vi "Keithley 2400 - Controle Fonte.vi"() -> ()   [LabVIEW 2011]
uses:
  <vilib>/Utility/file.llb/Write To Spreadsheet File (DBL).vi
panel:
  out "XY Graph":T1(graph)
  in  "VoltVector":dbl[](array[numeric])
  out "V(log)xI(log)":cluster{"Y":dbl[], "Y":dbl[]}[](graph)
  in  "Arquivo:":path=path "c:/dados.txt"
  in  "Corrente início:":dbl
  in  "CurrVector":dbl[](array[numeric])
  out "VxI":cluster{"Y":dbl[], "Y":dbl[]}[](graph)
  out "Corrente:":dbl
  out "Tensão:":dbl
  in  "Corrente limite (A):":dbl=2e-06
  in  "Porta Keithley:":refnum<visa-resource-name>="COM5"
  in  "Tensão passo (V):":dbl=1.0
  in  "Tensão final (V):":dbl=5.0
  in  "Tensão inicial (V):":dbl=1.0 caption="Tensão início:"
  in  "Medir":bool
  in  "Número de medidas:":i32=5
  in  "stop":bool
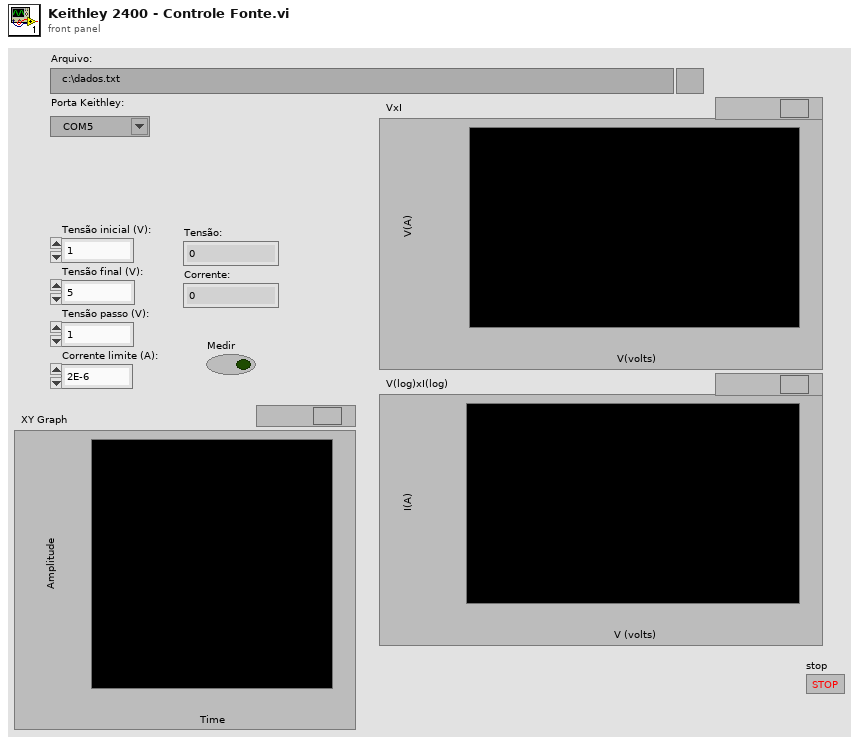
[diagram p1: front panel]
types:
  T1 = cluster{"VoltVector":dbl[], "CurrVector":dbl[]}[]
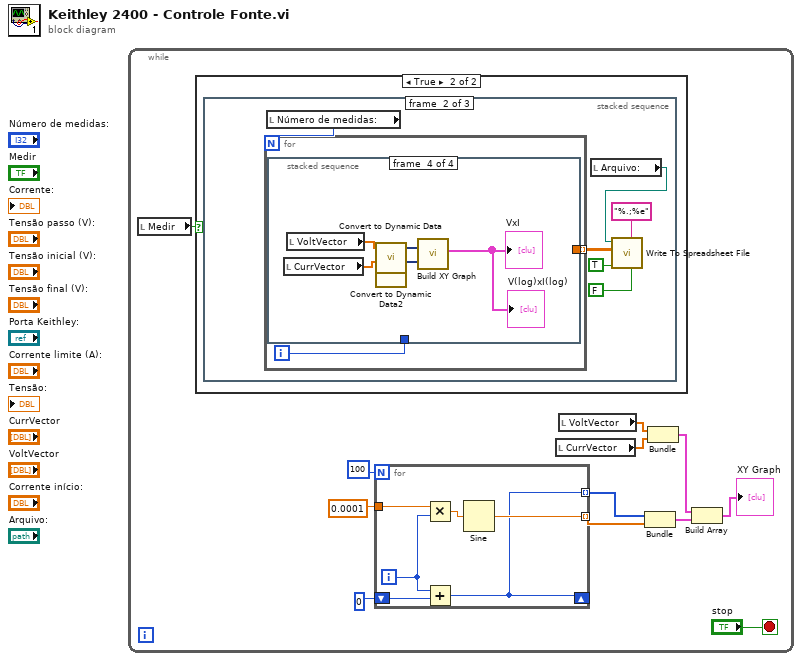
[diagram p0: block diagram]
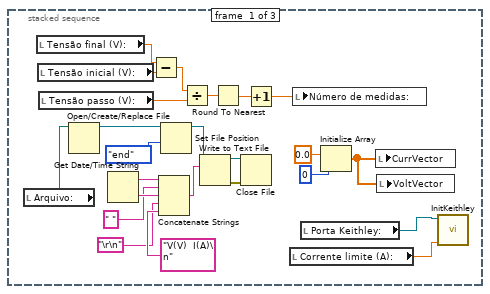
[diagram p3: hidden frame]
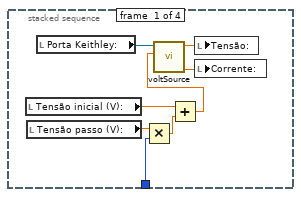
[diagram p4: hidden frame]
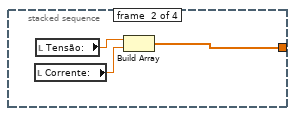
[diagram p5: hidden frame]
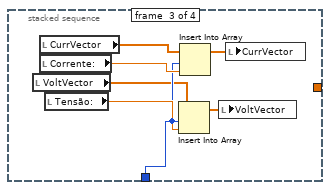
[diagram p6: hidden frame]
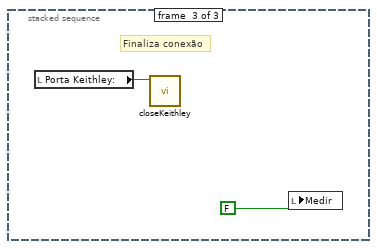
[diagram p7: hidden frame]
diagram:
  n1 = while {
    stop <- "stop" stop-if-true
    n2 = local read "Medir"() -> (w11:bool)
    n3 = case shown="True" w11 {
      frame False {
      }
      frame True {
        n4 = stacked-sequence {
          frame #0 {
            n5 = local read "Arquivo:"() -> (w23:path)
            n6 = local read "Tensão final (V):"() -> (w38:dbl)
            n7 = local read "Tensão inicial (V):"() -> (w39:dbl)
            n8 = local read "Tensão passo (V):"() -> (w41:dbl)
            n9 = Open/Create/Replace File(file path (use dialog)=w23) -> (refnum out=w24:refnum<file>)  [unwired: 5 in, 2 out]
            n10 = Get Date/Time String() -> (date string=w31:string, time string=w29:string)  [unwired: 3 in]
            n11 = Subtract(x=w38, y=w39) -> (x-y=w40:dbl)
            n12 = Concatenate Strings(w31, " " ("string"), w29, "\r\n", "V(V)  I(A)\n" ("text")) -> (w30:string)
            n13 = Set File Position(refnum=w24, from (0:start)=enum16{"start", "end", "current"}."end") -> (refnum out=w26:refnum<file>)  [unwired: 2 in, 1 out]
            n14 = Divide(x=w40, y=w41) -> (x/y=w42:dbl)
            n15 = Write to Text File(file (use dialog)=w26, text=w30) -> (refnum out=w32:refnum<file>, error out=w33:errorcluster)  [unwired: 2 in, 1 out]
            n16 = Round To Nearest(number=w42) -> (nearest integer value=w36:dbl)
            n17 = Close File(refnum=w32, error in=w33) -> ()  [unwired: 2 out]
            n18 = Increment(x=w36) -> (x+1=w37:dbl)
            n19 = local read "Corrente limite (A):"() -> (w21:dbl)
            n20 = local write "Número de medidas:"(w37) -> ()
            n21 = local read "Porta Keithley:"() -> (w22:refnum<visa-resource-name>)
            n22 = Initialize Array(0.0 ("element"), 0 ("dimension size")) -> (w20:dbl[])
            n23 = local write "CurrVector"(w20) -> ()
            n24 = local write "VoltVector"(w20) -> ()
            n25 = call "InitKeithley.vi"("limite:"=w21, "Porta:"=w22) -> ()  [unwired: 10 in]
          }
          frame #1 {
            n26 = local read "Número de medidas:"() -> (w48:i32)
            n27 = for {
              N: w48 -> [_]
              tunnel: [w49] -> w45 mode=indexing
              i -> [w50]
              n28 = stacked-sequence {
                tunnel: w50 -> [w55 _ w66 _]
                tunnel: [_ w61 _ _] -> w49
                frame #0 {
                  n29 = local read "Tensão inicial (V):"() -> (w57:dbl)
                  n30 = local read "Tensão passo (V):"() -> (w56:dbl)
                  n31 = local read "Porta Keithley:"() -> (w58:refnum<visa-resource-name>)
                  n32 = Multiply(x=w56, y=w55) -> (x*y=w54:dbl)
                  n33 = Add(x=w57, y=w54) -> (x+y=w53:dbl)
                  n34 = call "voltSource.vi"("Tensão aplicada:"=w53, "Porta:"=w58) -> ("Corrente:"=w51:dbl, "Tensão:"=w52:dbl)  [unwired: 8 in]
                  n35 = local write "Tensão:"(w52) -> ()
                  n36 = local write "Corrente:"(w51) -> ()
                }
                frame #1 {
                  n37 = local read "Corrente:"() -> (w59:dbl)
                  n38 = local read "Tensão:"() -> (w60:dbl)
                  n39 = Build Array(w60, w59) -> (w61:dbl[])
                }
                frame #2 {
                  n40 = local read "VoltVector"() -> (w63:dbl[])
                  n41 = local read "CurrVector"() -> (w62:dbl[])
                  n42 = local read "Corrente:"() -> (w68:dbl)
                  n43 = local read "Tensão:"() -> (w67:dbl)
                  n44 = Insert Into Array(array=w63, index=w66, new element=w67) -> (w64:dbl[])
                  n45 = Insert Into Array(array=w62, index=w66, new element=w68) -> (w65:dbl[])
                  n46 = local write "VoltVector"(w64) -> ()
                  n47 = local write "CurrVector"(w65) -> ()
                }
                frame #3 {
                  n48 = local read "CurrVector"() -> (w69:dbl[])
                  n49 = local read "VoltVector"() -> (w70:dbl[])
                  n50 = call "Convert to Dynamic Data"("Array"=w70) -> ("Dynamic Data Type"=w73:dynamicdata)  [unwired: 3 in]
                  n51 = call "Convert to Dynamic Data2"("Array"=w69) -> ("Dynamic Data Type"=w72:dynamicdata)  [unwired: 3 in]
                  n52 = call "Build XY Graph"("Y Input"=w72, "X Input"=w73) -> ("XY Graph"=→"VxI" →"V(log)xI(log)":cluster{"Y":dbl[], "Y":dbl[]}[])  [unwired: 3 in, 6 out]
                }
              }
            }
            n53 = local read "Arquivo:"() -> (w43:path)
            n54 = call-poly <vilib>:"Write To Spreadsheet File.vi"("transpose? (no:F)"=FALSE, "format (%.3f)"="%.;%e", "append to file? (new file:F)"=TRUE, "2D data"=w45, "file path (dialog if empty)"=w43) -> ()  [unwired: 3 in, 1 out]
          }
          frame #2 {
            # "Finaliza conexão"
            n55 = local read "Porta Keithley:"() -> (w74:refnum<visa-resource-name>)
            n56 = call "closeKeithley.vi"("Porta:"=w74) -> ()  [unwired: 11 in]
            n57 = local write "Medir"(FALSE ("Medir")) -> ()
          }
        }
      }
    }
    n58 = for {
      N: 100 -> [_]
      shift-right: [w14] -> _
      shift-left: 0 -> [w18]
      tunnel: [w16] -> w2 mode=indexing
      tunnel: [w14] -> w3 mode=indexing
      tunnel: 0.0001 -> [w13]
      i -> [w17]
      n59 = Multiply(x=w13, y=w17) -> (x*y=w15:dbl)
      n60 = Add(x=w17, y=w18) -> (x+y=w14:i32)
      n61 = Sine(x=w15) -> (sin(x)=w16:dbl)
    }
    n62 = local read "CurrVector"() -> (w9:dbl[])
    n63 = local read "VoltVector"() -> (w10:dbl[])
    n64 = Bundle "Bundle"(w3, w2) -> (w4:cluster{i32[], dbl[]})  [unwired: 1 in]
    n65 = Bundle("VoltVector"=w10, "CurrVector"=w9) -> (w5:cluster{"VoltVector":dbl[], "CurrVector":dbl[]})  [unwired: 1 in]
    n66 = Build Array(w5, w4) -> (→"XY Graph":T1)
  }
